vi "Icon_Fill in Body.vi"(6 "Body Rectangle":T3={"Region"={"Left"=0, "Top"=0, "Right"=0, "Bottom"=0, "Width"=0, "Height"=0, "Start"={"Left"=0, "Top"=0}}, "Color"=7, "Fill?"=TRUE}, 8 "Error":errorcluster, 11 "ICON Cluster":T6={"Header"="", "Body"=[], "ImageData"={"image type"=0, "image depth"=0, "image"=[], "mask"=[], "colors"=[], "Rectangle"={"left"=0, "top"=0, "right"=0, "bottom"=0}}, "New Icon"=bytes[0], "Line Status"=[], "Format"={"Color"={"Body txt"=255, "Body Back"=12632256, "Frame"=0, "Header txt"=32768, "Header Back"=16744703, "type"=enum."2 Color"}, "Icon Sizing"={"Rule"=enum."Static", "Header"=TRUE, "Rows"=5, "Width"=32, "Position"=enum."MID-CTR"}}} {"Format"."Icon Sizing"."Rows" min=1 max=5 step=1; "Format"."Icon Sizing"."Width" min=7 max=32 step=1}) -> (0 "Error Out":errorcluster, 3 "ICON Cluster Out":T6={"Header"="", "Body"=[], "ImageData"={"image type"=0, "image depth"=0, "image"=[], "mask"=[], "colors"=[], "Rectangle"={"left"=0, "top"=0, "right"=0, "bottom"=0}}, "New Icon"=bytes[0], "Line Status"=[], "Format"={"Color"={"Body txt"=255, "Body Back"=12632256, "Frame"=0, "Header txt"=32768, "Header Back"=16744703, "type"=enum."2 Color"}, "Icon Sizing"={"Rule"=enum."Static", "Header"=TRUE, "Rows"=5, "Width"=32, "Position"=enum."MID-CTR"}}} {"Format"."Icon Sizing"."Rows" min=1 max=5 step=1; "Format"."Icon Sizing"."Width" min=7 max=32 step=1}, 5 "Data Array Out":T1[](array[typedef]))   [LabVIEW 2009]
doc: "Draws body text in icon"
uses:
  Controls/Cluster/Cluster_Icon Data.ctl
  Controls/String_Picture/STRING_Line Display.ctl
  Controls/Array/String Array_Body Text.ctl
  Controls/Cluster/Cluster_Image Data.ctl
  Controls/Cluster/CLuster_Selectoin Box.ctl
  Controls/String_Picture/Picture_Icon.ctl
  Controls/Cluster/Cluster_Icon Format.ctl
  Controls/Cluster/Cluster_Icon Color Set.ctl
  Controls/Enum/ENUM_Frame Template Select.ctl
  Controls/Cluster/Cluster_Sizing Data.ctl
  Controls/Enum/ENUM_Icon Sizing.ctl
  Controls/Enum/RBENUM_Icon Position.ctl
  Controls/Cluster/Cluster_BOX Data.ctl
  Controls/Cluster/Cluster_Region info.ctl
  Controls/Cluster/Cluster_Top Left position.ctl
  Controls/Cluster/CLuster_Line Fit Results.ctl
  Controls/Enum/ENUM RB_Fit Result.ctl
  Controls/Cluster/Cluster_Text Color Set.ctl
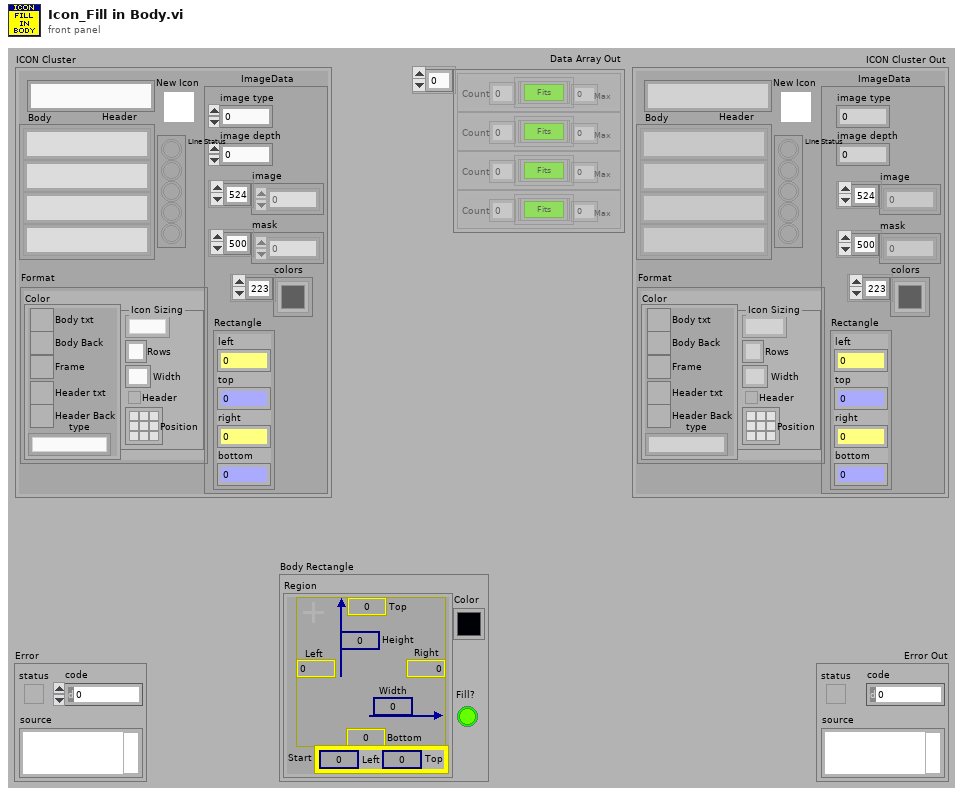
[diagram p1: front panel]
types:
  T1 = typedef "CLuster_Line Fit Results.ctl" = cluster{"Fit Result":T2, "Max":i32, "Count":i32}
  T2 = typedef "ENUM RB_Fit Result.ctl" = enum32{"Fits", "Almost Fits", "NO Fit"}
  T3 = typedef "Cluster_BOX Data.ctl" = cluster{"Region":T4, "Color":u32, "Fill?":bool}
  T4 = typedef "Cluster_Region info.ctl" = cluster{"Left":i32, "Top":i32, "Right":i32, "Bottom":i32, "Width":u32, "Height":u32, "Start":T5}
  T5 = typedef "Cluster_Top Left position.ctl" = cluster{"Left":i32, "Top":i32}
  T6 = typedef "Cluster_Icon Data.ctl" = cluster{"Header":T7, "Body":T8, "ImageData":T9, "New Icon":T11, "Line Status":bool[], "Format":T12}
  T7 = typedef "STRING_Line Display.ctl" = string
  T8 = typedef "String Array_Body Text.ctl" = T7[]
  T9 = typedef "Cluster_Image Data.ctl" = cluster{"image type":i32, "image depth":i32, "image":u8[], "mask":u8[], "colors":u32[], "Rectangle":T10}
  T10 = typedef "CLuster_Selectoin Box.ctl" = cluster{"left":i16, "top":i16, "right":i16, "bottom":i16}
  T11 = typedef "Picture_Icon.ctl" = picture
  T12 = typedef "Cluster_Icon Format.ctl" = cluster{"Color":T13, "Icon Sizing":T15}
  T13 = typedef "Cluster_Icon Color Set.ctl" = cluster{"Body txt":u32, "Body Back":u32, "Frame":u32, "Header txt":u32, "Header Back":u32, "type":T14}
  T14 = typedef "ENUM_Frame Template Select.ctl" = enum16{"2 Color", "5 Color"}
  T15 = typedef "Cluster_Sizing Data.ctl" = cluster{"Rule":T16, "Header":bool, "Rows":u32, "Width":u32, "Position":T17}
  T16 = typedef "ENUM_Icon Sizing.ctl" = enum16{"Static", "Auto"}
  T17 = typedef "RBENUM_Icon Position.ctl" = enum32{"LFT-TOP", "MID-TOP", "RGT-TOP", "LFT-CTR", "MID-CTR", "RGT-CTR", "LFT-BOT", "MID-BOT", "RGT-BOT"}
  T18 = typedef "Cluster_Text Color Set.ctl" = cluster{"BG":u32, "FG":u32}
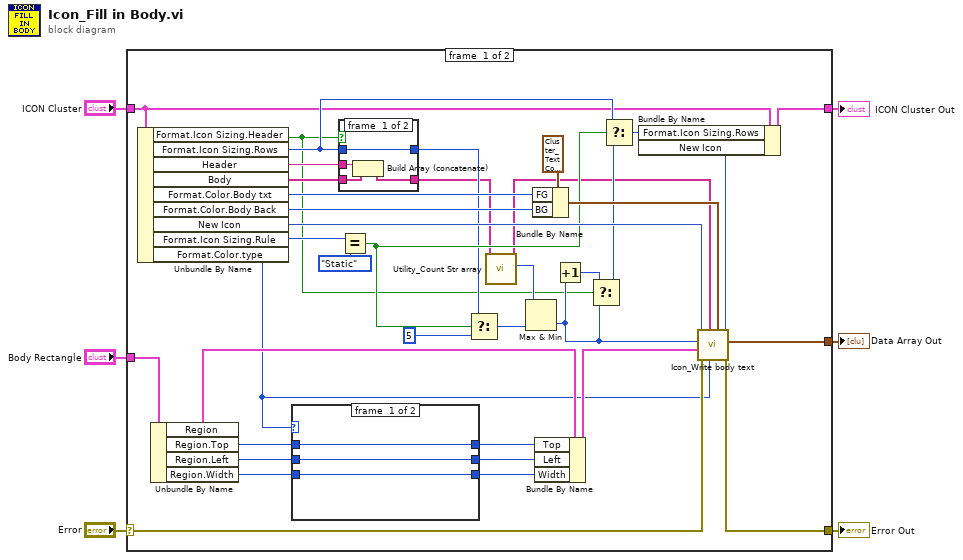
[diagram p0: block diagram]
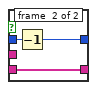
[diagram p2: hidden frame]
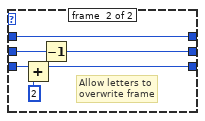
[diagram p3: hidden frame]
diagram:
  n1 = case shown="No Error" "Error" {
    selector: "Error" -> [w36 w61]
    tunnel: "ICON Cluster" -> [w9 w62]
    tunnel: [w44 w62] -> w5
    tunnel: [w18 w61] -> w4
    tunnel: "Body Rectangle" -> [w24 _]
    tunnel: [w41 _] -> w2
    frame #0 {
      n2 = Unbundle By Name(w9) -> ("Format.Icon Sizing.Header"=w12:bool, "Format.Icon Sizing.Rows"=w13:u32, "Header"=w15:T7, "Body"=w14:T8, "Format.Color.Body txt"=w38:u32, "Format.Color.Body Back"=w39:u32, "New Icon"=w43:T11, "Format.Icon Sizing.Rule"=w32:T16, "Format.Color.type"=w11:T14)
      n3 = Unbundle By Name(w24) -> ("Region"=w23:T4, "Region.Top"=w25:i32, "Region.Left"=w35:i32, "Region.Width"=w34:u32)
      n4 = case shown="\"2 Color\"" w11 {
        tunnel: w35 -> [w54 w60]
        tunnel: [w53 w59] -> w19
        tunnel: [w54 w58] -> w20
        tunnel: w34 -> [w53 w57]
        tunnel: w25 -> [w52 w55]
        tunnel: [w52 w55] -> w21
        frame #0 {
        }
        frame #1 {
          # "Allow letters to \noverwrite frame"
          n5 = Add(x=w57, y=u32 2 ("x")) -> (x+y=w59:u32)
          n6 = Decrement(x=w60) -> (x-1=w58:i32)
        }
      }
      n7 = case shown="True" w12 {
        tunnel: [w45 w51] -> w7
        tunnel: w14 -> [w46 w51]
        tunnel: w13 -> [w48 w50]
        tunnel: [w48 w49] -> w17
        tunnel: w15 -> [w47 _]
        frame #0 {
          n8 = Build Array (concatenate)(w47, w46) -> (w45:T8)
        }
        frame #1 {
          n9 = Decrement(x=w50) -> (x-1=w49:u32)
        }
      }
      n10 = Equal?(x=w32, y=ENUM_Icon_Sizing."Static") -> (x = y?=w28:bool)
      n11 = Select(t=w17, s=w28, f=u32 5) -> (s? t:f=w29:u32)
      n12 = call "Utility_Count Str array.vi"("String Array"=w7) -> ("Count Out"=w33:i16, "String Array Out"=w8:T8)  [unwired: 8 in, 1 out]
      n13 = Max & Min(x=w33, y=w29) -> (min(x,y)=w16:u32)  [unwired: 1 out]
      n14 = Bundle By Name(cluster=T18 {"BG"=128, "FG"=16764108} ("Color Set In"), "FG"=w38, "BG"=w39) -> (w37:T18)
      n15 = Bundle By Name(cluster=w23, "Top"=w21, "Left"=w20, "Width"=w19) -> (w22:T4)
      n16 = Increment(x=w16) -> (x+1=w27:u32)
      n17 = Select(t=w27, s=w12, f=w16) -> (s? t:f=w26:u32)
      n18 = Select(t=w13, s=w28, f=w26) -> (s? t:f=w10:u32)
      n19 = call "Icon_Write body text.vi"("Color Set"=w37, "Frame"=w11, "Text Array"=w8, "Error"=w36, "Region"=w22, "Line Count"=w16, "Icon"=w43) -> ("Error Out"=w18:errorcluster, "Result Array Out"=w41:T1[], "Icon Out"=w42:T11)  [unwired: 2 in]
      n20 = Bundle By Name(cluster=w9, "Format.Icon Sizing.Rows"=w10, "New Icon"=w42) -> (w44:T6)
    }
    frame #1 {
    }
  }
  "ICON Cluster Out" <- w5
  "Error Out" <- w4
  "Data Array Out" <- w2
